vi "Fit Cernox.vi"(7 "Calculate R in":dbl[](array[numeric]), 8 "error in":errorcluster, 9 "Polynomial order":i32=7, 10 "fit mode":T4(ring), 11 "Raw data source":T1={"File Path"=path "\\\\myhome\\NHMFLDATA/Data/PPMS/October_2025/102425/m001_164026_102425.tdms", "offset (0)"=3500, "count (-1: all)"=39500, "channel name(s) in"=["LakeShore 336 (12) A", "LakeShore 336 (12) B Raw"], "group"="p"}) -> (0 "error out":errorcluster, 1 "deviation":dbl[](array[numeric]), 2 "T subset":dbl[](graph), 3 "R":dbl[](array[numeric]), 4 "Fit  T":dbl[](array[numeric]), 5 "Calculated T out":dbl[](array[numeric]))   [LabVIEW 2025]
uses:
  <vilib>/Analysis/6fits.llb/Curve Fitting Criteria.ctl
  <vilib>/Analysis/6fits.llb/General Linear Fit Algorithm.ctl
  <vilib>/Analysis/polynomials.llb/1D Polynomial Evaluation (DBL).vi
  <vilib>/Analysis/NI_AALPro.lvlib
panel:
  out "T out":dbl
  in  "algorithm":T2 items=["SVD", "Givens", "Givens2", "Householder", "LU Decomposition", "Cholesky", "SVD for Rank Deficient H"]
  in  "method":T3 items=["Least Square", "Least Absolute Residual", "Bisquare"]
  out "Difference":cluster{dbl[], dbl[]}[](graph)
  out "residue":dbl
  in  "R column":i32=1
  in  "T column":i32
  out "Fit coef":dbl[](array[numeric]) format="%+#_18g"
  out "Linear Graph":cluster{dbl[], dbl[]}[](graph)
  out "Log Graph":cluster{dbl[], dbl[]}[](graph)
  out "Input data":dbl[][](array[numeric])
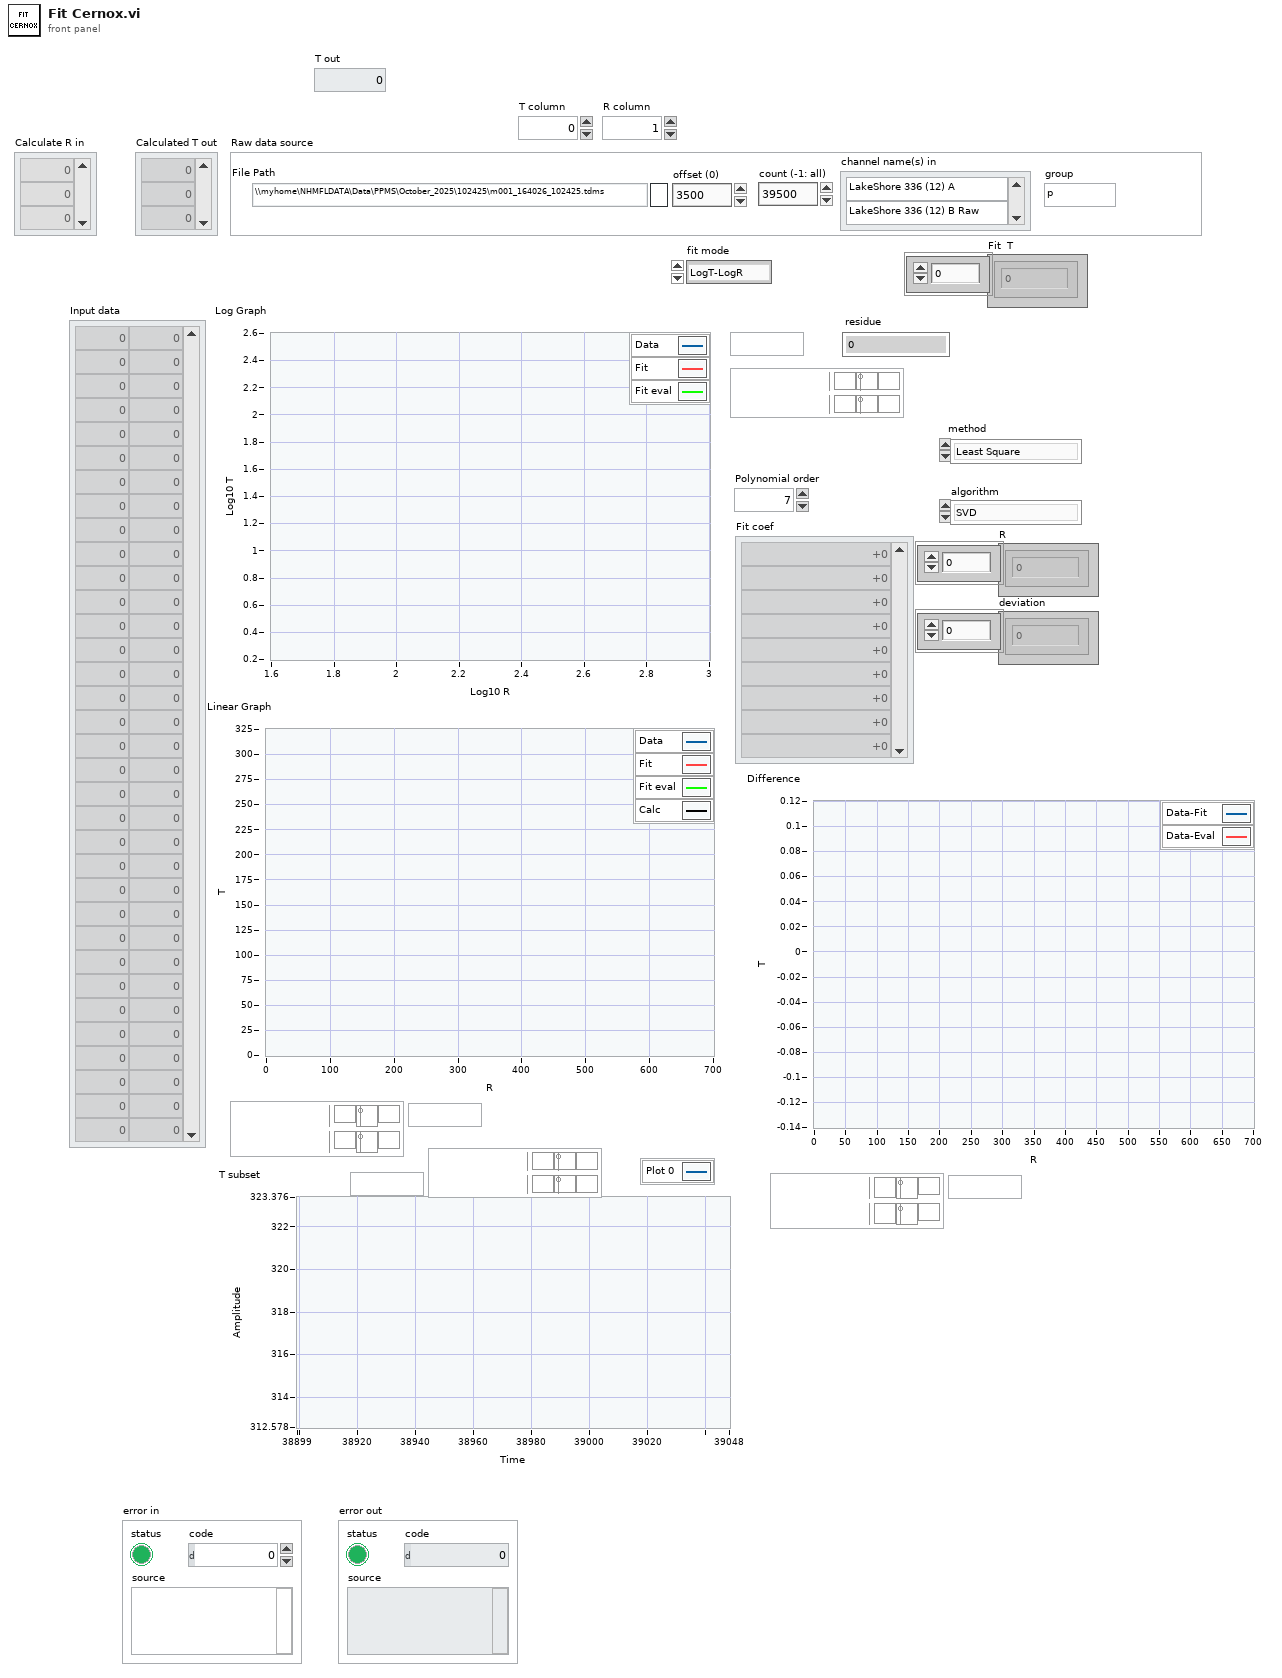
[diagram p1: front panel]
types:
  T1 = cluster{"File Path":path, "offset (0)":i64, "count (-1: all)":i64, "channel name(s) in":string[], "group":string}
  T2 = typedef "NI_AALPro.lvlib/General Linear Fit Algorithm.ctl" = u16
  T3 = typedef "NI_AALPro.lvlib/Curve Fitting Criteria.ctl" = u16
  T4 = enum16{"LogT-LogR", "T-LogR", "T-R", "T-1/R", "LogT-1/R"}
  T5 = enum16{"open", "open or create", "create or replace", "create", "open (read-only)"}
  T6 = cluster{"all rows":dbl[], "Best Polynomial Fit":dbl[]}
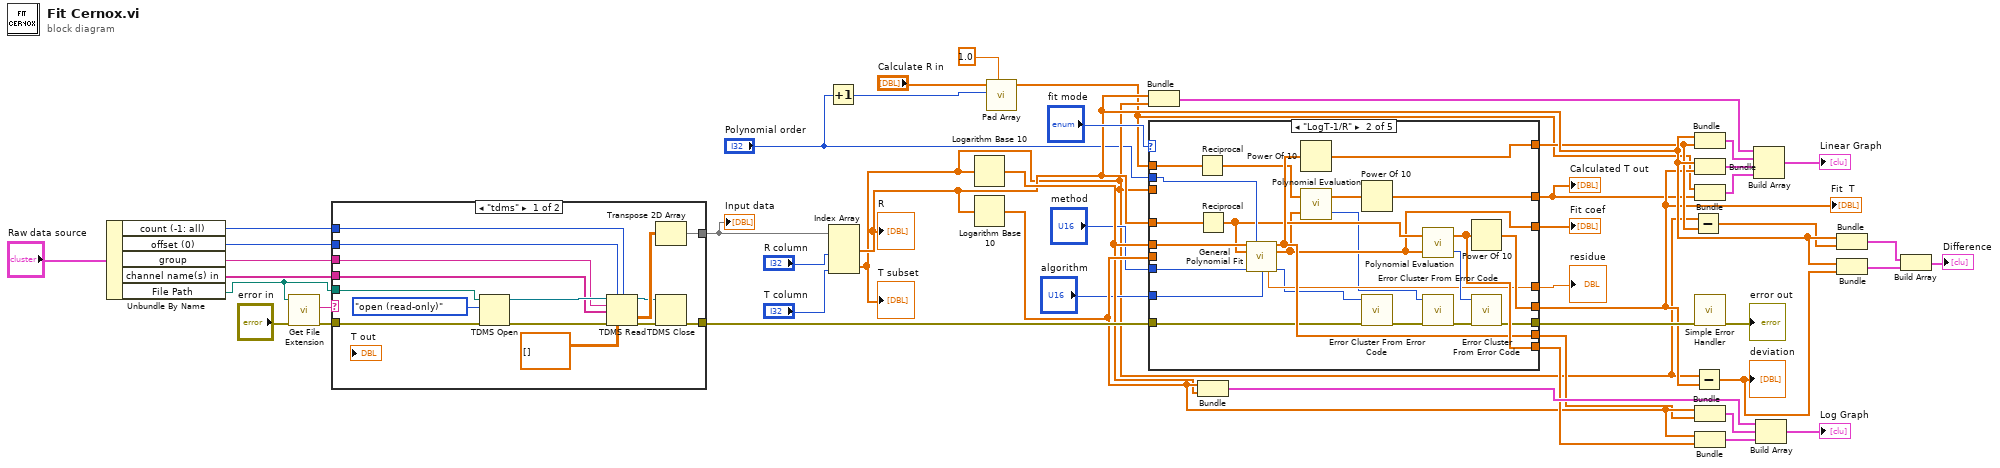
[diagram p0: block diagram]
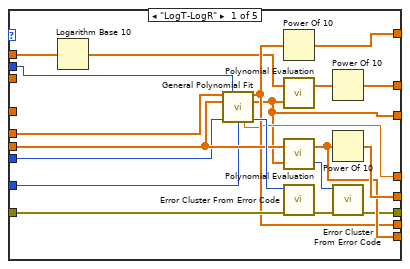
[diagram p2: hidden frame]
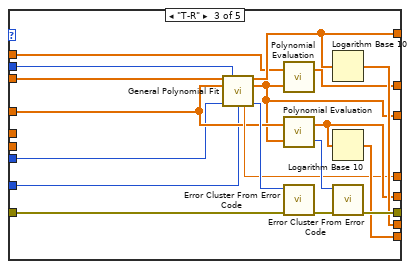
[diagram p3: hidden frame]
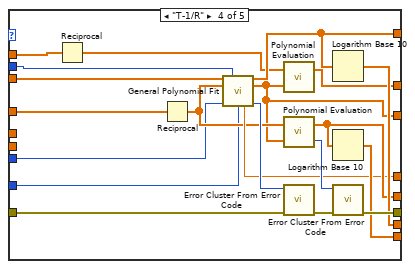
[diagram p4: hidden frame]
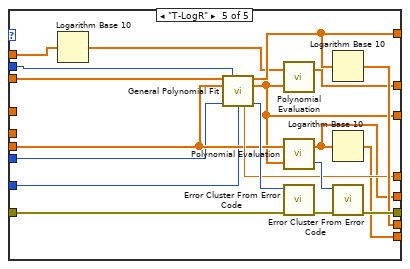
[diagram p5: hidden frame]
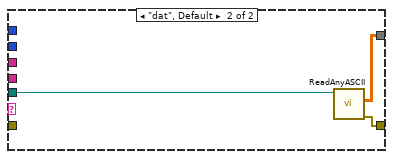
[diagram p6: hidden frame]
diagram:
  n1 = Unbundle By Name("Raw data source") -> ("count (-1: all)"=w9:i64, "offset (0)"=w10:i64, "group"=w8:string, "channel name(s) in"=w11:string[], "File Path"=w12:path)
  n2 = call <vilib>:"Get File Extension.vi"("error in (no error)"="error in", "file"=w12) -> ("error out"=w15:errorcluster, "lowercase file extension"=w35:string)  [unwired: 5 in, 3 out]
  n3 = case shown="\"tdms\"" w35 {
    tunnel: [w55 w66] -> w41
    tunnel: w12 -> [w63 w65]
    tunnel: [w54 w64] -> w34
    tunnel: w15 -> [w53 _]
    tunnel: w11 -> [w52 _]
    tunnel: w10 -> [w51 _]
    tunnel: w9 -> [w50 _]
    tunnel: w8 -> [w49 _]
    frame "tdms" {
      n4 = TDMS Open(8:w53, 10:T5."open (read-only)" ("operation (0:open)"), 11:w63) -> (0:w60:errorcluster, 3:w61:refnum<k34>)  [unwired: 4 in]
      n5 = TDMS Read(0:w61, 1:w51, 2:w50, 5:w49, 7:w52, 11:w60, 12:dbl[][] []) -> (4:w56:refnum<k34>, 10:w58:dbl[][], 15:w57:errorcluster)  [unwired: 1 in, 3 out]
      n6 = Transpose 2D Array(2D array=w58) -> (transposed array=w55:dbl[][])
      n7 = TDMS Close(8:w57, 11:w56) -> (0:w54:errorcluster)  [unwired: 1 out]
    }
    frame "dat", Default {
      n8 = call "ReadAnyASCII.vi"("file path (dialog if empty)"=w65) -> ("error out"=w64:errorcluster, "all rows"=w66:dbl[][])  [unwired: 8 in, 1 out]
    }
  }
  "Input data" <- w41
  n9 = Increment(x="Polynomial order") -> (x+1=w4:i32)
  n10 = Index Array(array=w41, index (col) #1="R column", index (col) #2="T column") -> (element #1=w27:dbl[], element #2=w17:dbl[])  [unwired: 2 in]
  "T subset" <- w17
  "R" <- w27
  n11 = Logarithm Base 10(1:w17) -> (0:w32:dbl[])
  n12 = Logarithm Base 10(1:w27) -> (0:w33:dbl[])
  n13 = call "Pad Array.vi"("default element"=1.0, "Desired size"=w4, "Signal in"="Calculate R in") -> ("Signal out"=w2:dbl[])  [unwired: 8 in]
  n14 = Bundle("all rows"=w27, "all rows"=w17) -> (w42:cluster{"all rows":dbl[], "all rows":dbl[]})  [unwired: 1 in]
  n15 = case shown="\"LogT-1/R\"" "fit mode" {
    tunnel: "Polynomial order" -> [w86 w109 w127 w147 w166]
    tunnel: [w84 w108 w120 w140 w159] -> w26
    tunnel: [w83 w107 w118 w138 w155] -> w23
    tunnel: [w82 w106 w117 w137 w154] -> w39
    tunnel: [w69 w94 w111 w129 w149] -> w38
    tunnel: w34 -> [w81 w90 w125 w145 w164]
    tunnel: w33 -> [w80 _ _ _ w156]
    tunnel: w32 -> [w79 w105 _ _ _]
    tunnel: [w77 w103 w123 w143 w162] -> w31
    tunnel: [w75 w101 w119 w139 w158] -> w30
    tunnel: w27 -> [_ w97 w115 w135 _]
    tunnel: w17 -> [_ _ w121 w141 w160]
    tunnel: [w74 w100 w116 w136 w157] -> w28
    tunnel: "method" -> [w73 w99 w113 w133 w153]
    tunnel: "algorithm" -> [w72 w98 w114 w132 w152]
    tunnel: w2 -> [w71 w95 w112 w130 w151]
    tunnel: [w67 w91 w110 w128 w148] -> w7
    frame "LogT-LogR" {
      n16 = Logarithm Base 10(1:w71) -> (0:w70:dbl[])
      n17 = call <vilib>:"General Polynomial Fit.vi"("Y"=w79, "polynomial order"=w86, "X"=w80, "method"=w73, "algorithm"=w72) -> ("Best Polynomial Fit"=w75:dbl[], "Polynomial Coefficients"=w69:dbl[], "residue"=w74:dbl, "error"=w85:i32)  [unwired: 7 in]
      n18 = Power Of 10(x=w75) -> (10^x=w84:dbl[])
      n19 = call-poly <vilib>:"Polynomial Evaluation.vi"("P(x)"=w69, "A"=w70) -> ("P(A)"=w68:dbl[])  [unwired: 1 out]
      n20 = call-poly <vilib>:"Polynomial Evaluation.vi"("P(x)"=w69, "A"=w80) -> ("error"=w76:i32, "P(A)"=w82:dbl[])
      n21 = call <vilib>:"Error Cluster From Error Code.vi"("error in (no error)"=w81, "error code (0)"=w85) -> ("error out"=w78:errorcluster)  [unwired: 7 in]
      n22 = Power Of 10(x=w68) -> (10^x=w67:dbl[])
      n23 = Power Of 10(x=w82) -> (10^x=w83:dbl[])
      n24 = call <vilib>:"Error Cluster From Error Code.vi"("error in (no error)"=w78, "error code (0)"=w76) -> ("error out"=w77:errorcluster)  [unwired: 7 in]
    }
    frame "LogT-1/R" {
      n25 = Reciprocal(x=w95) -> (1/x=w93:dbl[])
      n26 = Reciprocal(x=w97) -> (1/x=w96:dbl[])
      n27 = call <vilib>:"General Polynomial Fit.vi"("Y"=w105, "polynomial order"=w109, "X"=w96, "method"=w99, "algorithm"=w98) -> ("Best Polynomial Fit"=w101:dbl[], "Polynomial Coefficients"=w94:dbl[], "residue"=w100:dbl, "error"=w88:i32)  [unwired: 7 in]
      n28 = Power Of 10(x=w101) -> (10^x=w108:dbl[])
      n29 = call-poly <vilib>:"Polynomial Evaluation.vi"("P(x)"=w94, "A"=w93) -> ("error"=w87:i32, "P(A)"=w92:dbl[])
      n30 = Power Of 10(x=w92) -> (10^x=w91:dbl[])
      n31 = call <vilib>:"Error Cluster From Error Code.vi"("error in (no error)"=w90, "error code (0)"=w88) -> ("error out"=w89:errorcluster)  [unwired: 7 in]
      n32 = call-poly <vilib>:"Polynomial Evaluation.vi"("P(x)"=w94, "A"=w96) -> ("error"=w102:i32, "P(A)"=w106:dbl[])
      n33 = call <vilib>:"Error Cluster From Error Code.vi"("error in (no error)"=w89, "error code (0)"=w87) -> ("error out"=w104:errorcluster)  [unwired: 7 in]
      n34 = Power Of 10(x=w106) -> (10^x=w107:dbl[])
      n35 = call <vilib>:"Error Cluster From Error Code.vi"("error in (no error)"=w104, "error code (0)"=w102) -> ("error out"=w103:errorcluster)  [unwired: 7 in]
    }
    frame "T-R" {
      n36 = call <vilib>:"General Polynomial Fit.vi"("Y"=w121, "polynomial order"=w127, "X"=w115, "method"=w113, "algorithm"=w114) -> ("Best Polynomial Fit"=w120:dbl[], "Polynomial Coefficients"=w111:dbl[], "residue"=w116:dbl, "error"=w126:i32)  [unwired: 7 in]
      n37 = call-poly <vilib>:"Polynomial Evaluation.vi"("P(x)"=w111, "A"=w112) -> ("P(A)"=w110:dbl[])  [unwired: 1 out]
      n38 = call-poly <vilib>:"Polynomial Evaluation.vi"("P(x)"=w111, "A"=w115) -> ("error"=w122:i32, "P(A)"=w118:dbl[])
      n39 = call <vilib>:"Error Cluster From Error Code.vi"("error in (no error)"=w125, "error code (0)"=w126) -> ("error out"=w124:errorcluster)  [unwired: 7 in]
      n40 = Logarithm Base 10(1:w120) -> (0:w119:dbl[])
      n41 = Logarithm Base 10(1:w118) -> (0:w117:dbl[])
      n42 = call <vilib>:"Error Cluster From Error Code.vi"("error in (no error)"=w124, "error code (0)"=w122) -> ("error out"=w123:errorcluster)  [unwired: 7 in]
    }
    frame "T-1/R" {
      n43 = Reciprocal(x=w130) -> (1/x=w131:dbl[])
      n44 = Reciprocal(x=w135) -> (1/x=w134:dbl[])
      n45 = call <vilib>:"General Polynomial Fit.vi"("Y"=w141, "polynomial order"=w147, "X"=w134, "method"=w133, "algorithm"=w132) -> ("Best Polynomial Fit"=w140:dbl[], "Polynomial Coefficients"=w129:dbl[], "residue"=w136:dbl, "error"=w146:i32)  [unwired: 7 in]
      n46 = call-poly <vilib>:"Polynomial Evaluation.vi"("P(x)"=w129, "A"=w131) -> ("P(A)"=w128:dbl[])  [unwired: 1 out]
      n47 = call-poly <vilib>:"Polynomial Evaluation.vi"("P(x)"=w129, "A"=w134) -> ("error"=w142:i32, "P(A)"=w138:dbl[])
      n48 = call <vilib>:"Error Cluster From Error Code.vi"("error in (no error)"=w145, "error code (0)"=w146) -> ("error out"=w144:errorcluster)  [unwired: 7 in]
      n49 = Logarithm Base 10(1:w140) -> (0:w139:dbl[])
      n50 = Logarithm Base 10(1:w138) -> (0:w137:dbl[])
      n51 = call <vilib>:"Error Cluster From Error Code.vi"("error in (no error)"=w144, "error code (0)"=w142) -> ("error out"=w143:errorcluster)  [unwired: 7 in]
    }
    frame "T-LogR" {
      n52 = Logarithm Base 10(1:w151) -> (0:w150:dbl[])
      n53 = call <vilib>:"General Polynomial Fit.vi"("Y"=w160, "polynomial order"=w166, "X"=w156, "method"=w153, "algorithm"=w152) -> ("Best Polynomial Fit"=w159:dbl[], "Polynomial Coefficients"=w149:dbl[], "residue"=w157:dbl, "error"=w165:i32)  [unwired: 7 in]
      n54 = call-poly <vilib>:"Polynomial Evaluation.vi"("P(x)"=w149, "A"=w150) -> ("P(A)"=w148:dbl[])  [unwired: 1 out]
      n55 = call-poly <vilib>:"Polynomial Evaluation.vi"("P(x)"=w149, "A"=w156) -> ("error"=w161:i32, "P(A)"=w155:dbl[])
      n56 = call <vilib>:"Error Cluster From Error Code.vi"("error in (no error)"=w164, "error code (0)"=w165) -> ("error out"=w163:errorcluster)  [unwired: 7 in]
      n57 = Logarithm Base 10(1:w159) -> (0:w158:dbl[])
      n58 = Logarithm Base 10(1:w155) -> (0:w154:dbl[])
      n59 = call <vilib>:"Error Cluster From Error Code.vi"("error in (no error)"=w163, "error code (0)"=w161) -> ("error out"=w162:errorcluster)  [unwired: 7 in]
    }
  }
  "Fit coef" <- w38
  "residue" <- w28
  "Calculated T out" <- w7
  "Fit  T" <- w23
  n60 = Bundle(w33, w32) -> (w48:cluster{dbl[], dbl[]})  [unwired: 1 in]
  n61 = Subtract(x=w17, y=w26) -> (x-y=w25:dbl[])
  n62 = Subtract(x=w17, y=w23) -> (x-y=w22:dbl[])
  "deviation" <- w22
  n63 = Bundle("all rows"=w27, "Best Polynomial Fit"=w26) -> (w43:T6)  [unwired: 1 in]
  n64 = Bundle("all rows"=w27, "P(A)"=w23) -> (w44:cluster{"all rows":dbl[], "P(A)":dbl[]})  [unwired: 1 in]
  n65 = Bundle("Signal out"=w2, "P(A)"=w7) -> (w6:cluster{"Signal out":dbl[], "P(A)":dbl[]})  [unwired: 1 in]
  n66 = call <vilib>:"Simple Error Handler.vi"("error in (no error)"=w31) -> ("error out"=→"error out":errorcluster)  [unwired: 4 in, 4 out]
  n67 = Bundle(w33, "Best Polynomial Fit"=w30) -> (w46:cluster{dbl[], "Best Polynomial Fit":dbl[]})  [unwired: 1 in]
  n68 = Bundle(w33, "P(A)"=w39) -> (w45:cluster{dbl[], "P(A)":dbl[]})  [unwired: 1 in]
  n69 = Build Array(w42, w43, w44, w6) -> (→"Linear Graph":cluster{"Signal out":dbl[], "P(A)":dbl[]}[])
  n70 = Build Array(w48, w46, w45) -> (→"Log Graph":cluster{dbl[], "P(A)":dbl[]}[])
  n71 = Bundle("all rows"=w27, w25) -> (w24:cluster{"all rows":dbl[], dbl[]})  [unwired: 1 in]
  n72 = Bundle("all rows"=w27, w22) -> (w21:cluster{"all rows":dbl[], dbl[]})  [unwired: 1 in]
  n73 = Build Array(w24, w21) -> (→"Difference":cluster{"all rows":dbl[], dbl[]}[])
